vi "MODBUS RTU Send Message.vi"(6 "Command (0)":u8, 7 "Unit Address (1)":u8, 8 "error in (no error)":errorcluster, 10 "Message (empty array)":u8[](array[numeric]), 11 "VISA session":refnum<visa-resource-name>) -> (0 "error out":errorcluster, 2 "Length Of Sent MSG":u8, 3 "dup VISA session":refnum<visa-resource-name>)   [LabVIEW 2017]
doc: "This VI sends the MODBUS message."
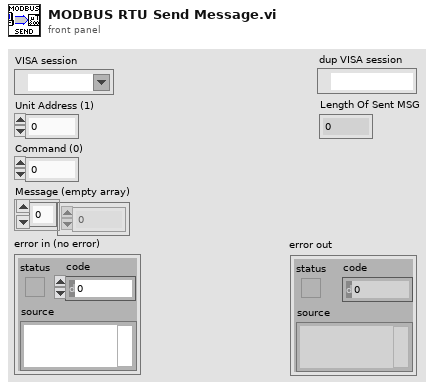
[diagram p1: front panel]
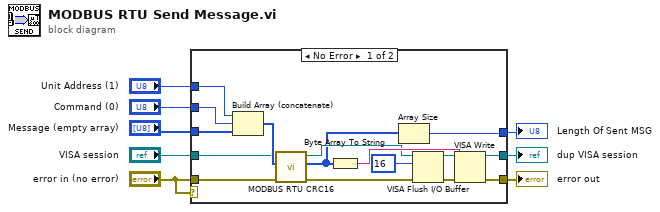
[diagram p0: block diagram]
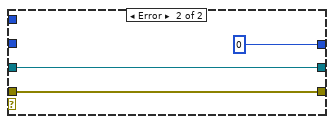
[diagram p2: hidden frame]
diagram:
  n1 = case shown="No Error" "error in (no error)" {
    tunnel: "error in (no error)" -> [w14 w26]
    tunnel: [w18 w26] -> w8
    tunnel: [w19 w27] -> w7
    tunnel: "Command (0)" -> [w24 _]
    tunnel: "Unit Address (1)" -> [w23 _]
    tunnel: "VISA session" -> [w12 w27]
    tunnel: [w22 0] -> w3
    tunnel: "Message (empty array)" -> [w21 _]
    frame No Error {
      n2 = Build Array (concatenate)(w23, w24, w21) -> (w13:u8[])
      n3 = call "MODBUS RTU CRC16.vi"("error in (no error)"=w14, "Message (empty array)"=w13, "VISA session"=w12) -> ("error out"=w11:errorcluster, "Message with CRC"=w9:u8[], "dup VISA session"=w10:refnum<visa-resource-name>)  [unwired: 5 in, 1 out]
      n4 = Byte Array To String(unsigned byte array=w9) -> (string=w20:string)
      n5 = Array Size(array=w9) -> (size(s)=w22:i32)
      n6 = VISA Flush I/O Buffer(VISA resource name=w10, mask (16)=u16 16, error in (no error)=w11) -> (VISA resource name out=w17:refnum<visa-resource-name>, error out=w16:errorcluster)
      n7 = VISA Write(VISA resource name=w17, write buffer=w20, error in (no error)=w16) -> (VISA resource name out=w19:refnum<visa-resource-name>, error out=w18:errorcluster)  [unwired: 1 out]
    }
    frame Error {
    }
  }
  "error out" <- w8
  "dup VISA session" <- w7
  "Length Of Sent MSG" <- w3
